vi "Selected Clock(Global Variable).vi"() -> ()   [LabVIEW 2020]
panel:
  out "Selected Alarm Clock":timestamp=timestamp(3671586000.8519278 s since 1904-01-01) format="%<%X\n%x>T"
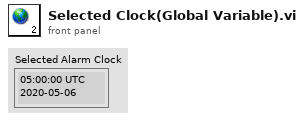
[diagram p1: front panel]
diagram:
